vi "GDSAPI_AddDesignPattern.vi"(8 "error in (no error)":errorcluster, 10 "InterfaceClass(*.lvclass)":path, 11 "ClassPath(*.lvclass)":path) -> (0 "error out":errorcluster)   [LabVIEW 2020]
doc: "This VI creates Methods in a class."
uses:
  <resource>/Framework/Providers/Open_GDS/ClassProviders/Provider_BaseClassInterface/BaseProvider_SubVIs/BaseProvider_DesignPatternsActions.ctl
  <resource>/Framework/Providers/Open_GDS/ClassProviders/DesignPatterns/Interface/Interface_SubVIs/InterfaceType.ctl
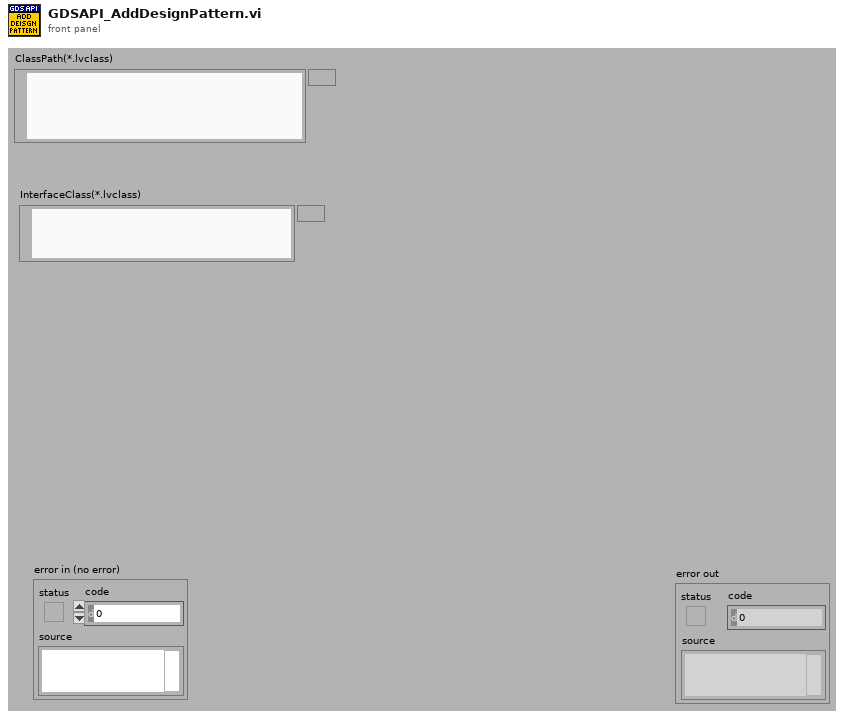
[diagram p1: front panel]
types:
  T1 = typedef "InterfaceType.ctl" = enum16{"ByAggregation", "ByViServer"}
  T2 = typedef "BaseProvider_DesignPatternsActions.ctl" = enum16{"AddPatternDialog", "GeneratePattern", "RemovePattern", "CreatePatternMethod", "UpdatePattern"}
  T3 = typedef "GDSLvCLass_ClassSettingsType.ctl" = cluster{"ClassProviderName":string, "ClassTemplateUsed":string, "ClassTemplateVersion":string, "ClassDescription":string, "PlugIns":T4[], "ConnectorPanePattern":string}
  T4 = typedef "GDSLvClass_PlugIn.ctl" = cluster{"Type":T5, "ID":string, "Version":string, "Path":path, "Name":string, "Data":variant}
  T5 = typedef "GDSLvClass_PlugInTypes.ctl" = enum16{"DesignPattern", "MethodTypes"}
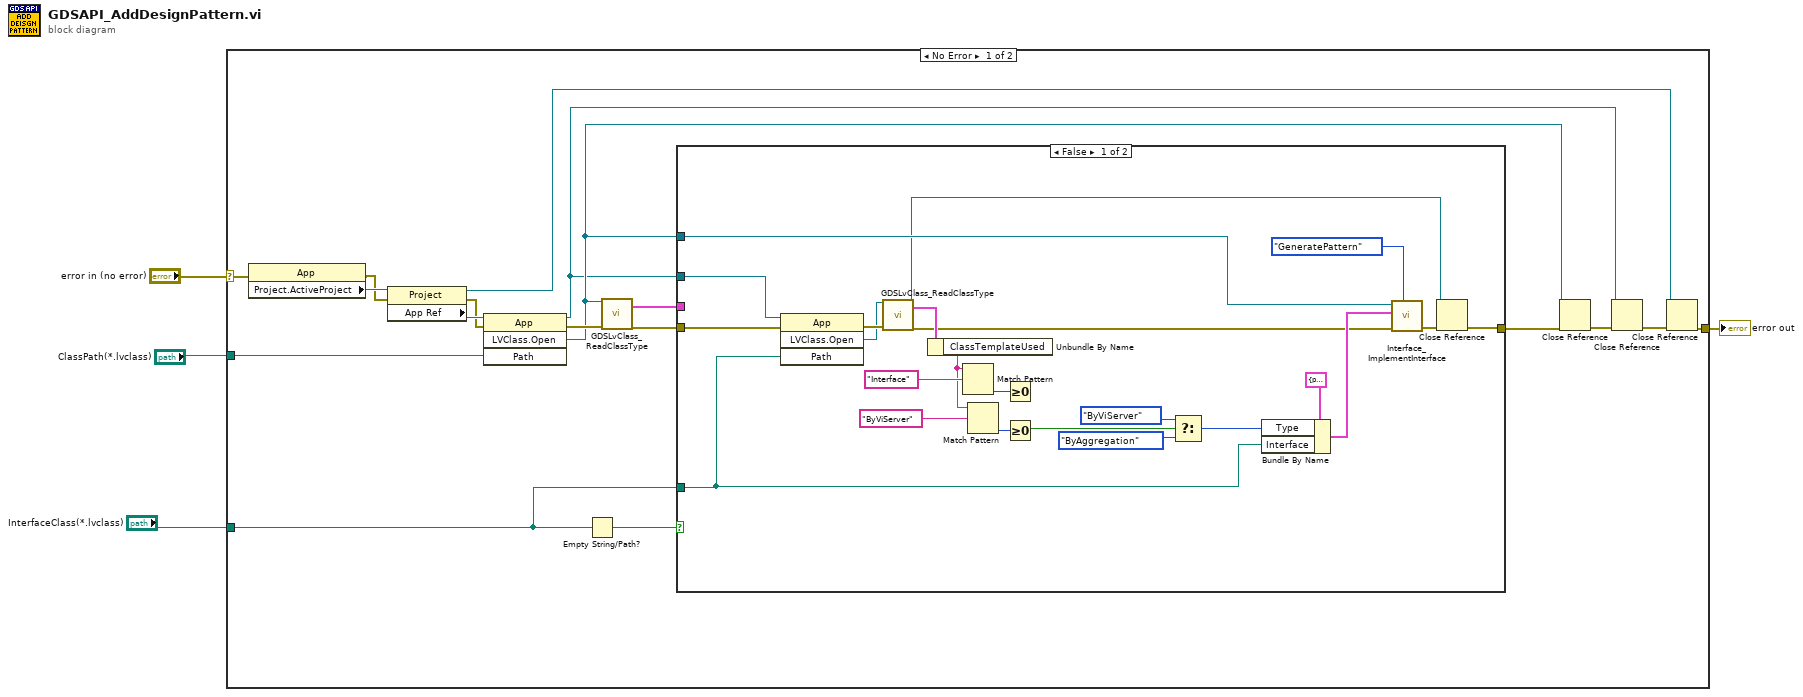
[diagram p0: block diagram]
diagram:
  n1 = case shown="No Error" "error in (no error)" {
    selector: "error in (no error)" -> [w5 w47]
    tunnel: "ClassPath(*.lvclass)" -> [w22 _]
    tunnel: [w15 w47] -> w3
    tunnel: "InterfaceClass(*.lvclass)" -> [w8 _]
    frame No Error {
      n2 = property class="App"(error in=w5) -> (error out=w18:errorcluster, "Project.ActiveProject"=w21:refnum<vi>)  [unwired: 1 in, 1 out]
      n3 = property class="Project"(reference=w21, error in=w18) -> (reference out=w11:refnum<vi>, error out=w19:errorcluster, "App Ref"=w20:refnum<vi>)
      n4 = invoke class="App" method="LVClass.Open"(reference=w20, error in=w19, "Path"=w22) -> (reference out=w6:refnum<vi>, error out=w14:errorcluster, "LVClass.Open"=w10:refnum<vi>)  [unwired: 1 in, 1 out]
      n5 = Empty String/Path?(string/path=w8) -> (empty?=w9:bool)
      n6 = call <resource>:"GDSLvClass_ReadClassType.vi"("Class Refnum In"=w10, "error in (no error)"=w14) -> ("ClassSettings"=w12:T3, "error out"=w13:errorcluster)  [unwired: 15 in, 1 out]
      n7 = case shown="False" w9 {
        tunnel: w13 -> [w33 w46]
        tunnel: w12 -> [_ _]
        tunnel: w10 -> [w34 _]
        tunnel: w8 -> [w28 _]
        tunnel: [w24 w46] -> w7
        tunnel: w6 -> [w32 _]
        frame False {
          n8 = invoke class="App" method="LVClass.Open"(reference=w32, error in=w33, "Path"=w28) -> (error out=w30:errorcluster, "LVClass.Open"=w29:refnum<vi>)  [unwired: 1 in, 2 out]
          n9 = call <resource>:"GDSLvClass_ReadClassType.vi"("Class Refnum In"=w29, "error in (no error)"=w30) -> ("Class Refnum Out"=w23:refnum<vi>, "ClassSettings"=w31:T3, "error out"=w26:errorcluster)  [unwired: 15 in]
          n10 = Unbundle By Name(w31) -> ("ClassTemplateUsed"=w41:string)
          n11 = Match Pattern(string=w41, regular expression="Interface") -> (offset past match=w42:i32)  [unwired: 1 in, 3 out]
          n12 = Match Pattern(string=w41, regular expression="ByViServer") -> (offset past match=w39:i32)  [unwired: 1 in, 3 out]
          n13 = Greater Or Equal To 0?(x=w42) -> ()  [unwired: 1 out]
          n14 = Greater Or Equal To 0?(x=w39) -> (x >= 0?=w38:bool)
          n15 = Select(t=InterfaceType."ByViServer" ("Type"), s=w38, f=InterfaceType."ByAggregation" ("Type")) -> (s? t:f=w27:T1)
          n16 = Bundle By Name(cluster=cluster{"Interface":path, "Type":T1} {"Interface"=path "", "Type"=enum."ByViServer"} ("DeisgnPatternData"), "Type"=w27, "Interface"=w28) -> (w35:cluster{"Interface":path, "Type":T1})
          n17 = call <resource>:"Interface_ImplementInterface.vi"("Action"=BaseProvider_DesignPatternsActions."GeneratePattern", "error in (no error)"=w26, "DataIn"=w35, "ClassRefToActOn"=w34) -> ("error out"=w25:errorcluster)  [unwired: 4 in, 3 out]
          n18 = Close Reference(reference=w23, error in (no error)=w25) -> (error out=w24:errorcluster)
        }
        frame True {
        }
      }
      n19 = Close Reference(reference=w10, error in (no error)=w7) -> (error out=w17:errorcluster)
      n20 = Close Reference(reference=w6, error in (no error)=w17) -> (error out=w16:errorcluster)
      n21 = Close Reference(reference=w11, error in (no error)=w16) -> (error out=w15:errorcluster)
    }
    frame Error {
    }
  }
  "error out" <- w3
